vi "(SubVI) stage readPI.vi"(3 "Axis":u32, 5 "read #":i32=7) -> (1 "position (um)":dbl)   [LabVIEW 2014]
uses:
  <vilib>/Analysis/baseanly.llb/Mean (DBL).vi
  <vilib>/Analysis/NI_AALBase.lvlib
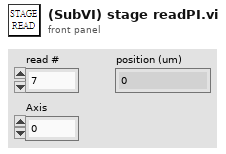
[diagram p1: front panel]
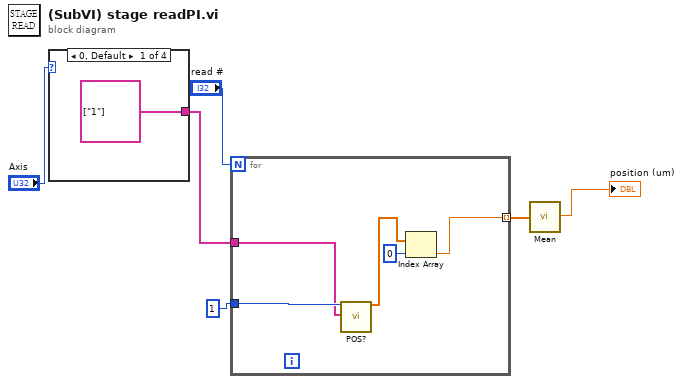
[diagram p0: block diagram]
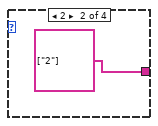
[diagram p2: hidden frame]
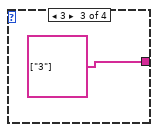
[diagram p3: hidden frame]
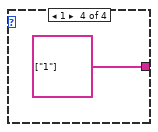
[diagram p4: hidden frame]
diagram:
  n1 = case shown="0, Default" "Axis" {
    tunnel: [string[] ["1"] string[] ["2"] string[] ["3"] string[] ["1"]] -> w2
    frame 0, Default {
    }
    frame 2 {
    }
    frame 3 {
    }
    frame 1 {
    }
  }
  n2 = for {
    N: "read #" -> [_]
    tunnel: 1 ("System no.") -> [w15]
    tunnel: w2 -> [w14]
    tunnel: [w11] -> w1 mode=indexing
    n3 = call "POS?.vi"("System no."=w15, "Axes to query"=w14) -> ("Position"=w13:dbl[])  [unwired: 16 in, 1 out]
    n4 = Index Array(array=w13, index=0) -> (element=w11:dbl)
  }
  n5 = call-poly <vilib>:"Mean.vi"("X"=w1) -> ("mean"=→"position (um)":dbl)  [unwired: 1 out]
